vi "loop deploy test.vi"() -> ()   [LabVIEW 2017, in "Routing and Faulting System Tests.lvclass"]
uses:
  Routing and Faulting System Tests.lvclass
panel:
  out "Open Error":errorcluster
  in  "error in":errorcluster
  out "error":bool
  out "error out":errorcluster
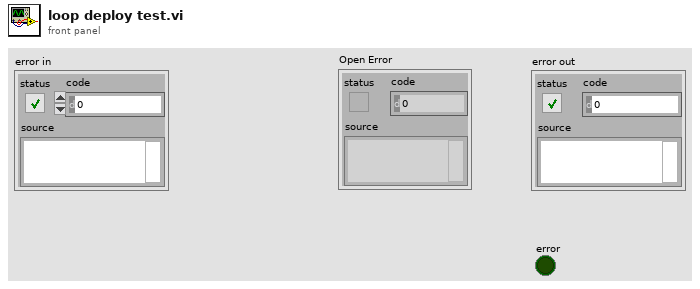
[diagram p1: front panel]
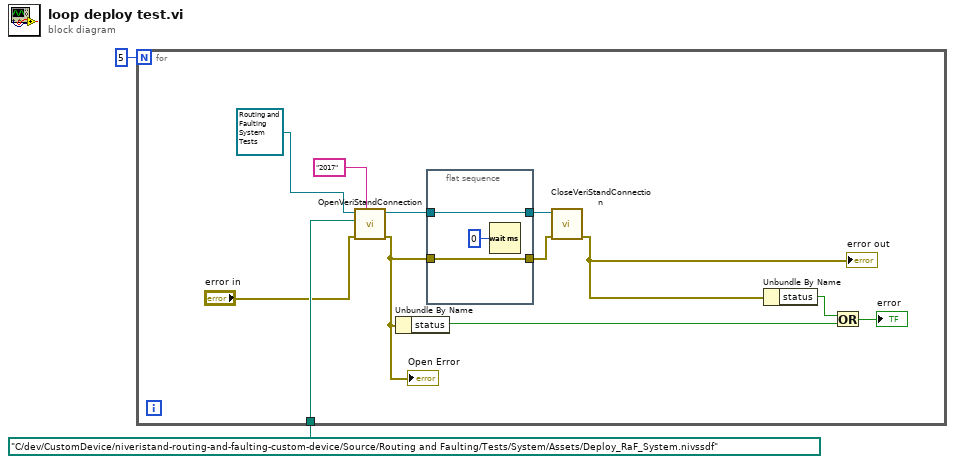
[diagram p0: block diagram]
diagram:
  n1 = for {
    N: 5 -> [_]
    tunnel: path "C:/dev/CustomDevice/niveristand-routing-and-faulting-custom-device/Source/Routing and Faulting/Tests/System/Assets/Deploy_RaF_System.nivssdf" ("System Definition File") -> [w9]
    n2 = call-dynamic "OpenVeriStandConnection.vi"("Minimum VeriStand Version (2015)"="2017", "error in (no error)"="error in", "System Definition File"=w9, "VeriStand Test Case in"=refnum<class "Routing and Faulting System Tests.lvclass"> refnum) -> ("error out"=w6:errorcluster, "VeriStand Test Case out"=w8:refnum<class "Routing and Faulting System Tests.lvclass">)  [unwired: 5 in, 1 out]
    "Open Error" <- w6
    n3 = Unbundle By Name(w6) -> ("status"=w11:bool)
    n4 = flat-sequence {
      tunnel: w8 -> [w16]
      tunnel: [w16] -> w7
      tunnel: w6 -> [w15]
      tunnel: [w15] -> w5
      frame #0 {
        n5 = Wait (ms)(milliseconds to wait=u32 0) -> ()  [unwired: 1 out]
      }
    }
    n6 = call-dynamic "CloseVeriStandConnection.vi"("error in (no error)"=w5, "VeriStand Test Case in"=w7) -> ("error out"=w3:errorcluster)  [unwired: 8 in, 1 out]
    "error out" <- w3
    n7 = Unbundle By Name(w3) -> ("status"=w12:bool)
    n8 = Or(x=w12, y=w11) -> (x .or. y?=→"error":bool)
  }
